vi "Tegam4040 - Close.vi"(8 "error in (no error)":errorcluster, 11 "Instrument Session Handle":u32 format="%x") -> (0 "error out":errorcluster)   [LabVIEW 2010, in "Tegam4040.lvlib"]
doc: "Closes a device session or event object specified by VISA resource name. For each VISA session that you open, you should close the session when you are finished with it. This function accepts all available classes."
uses:
  Tegam4040.lvlib
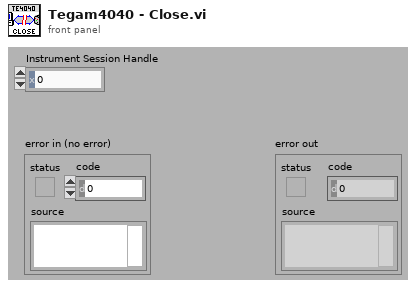
[diagram p1: front panel]
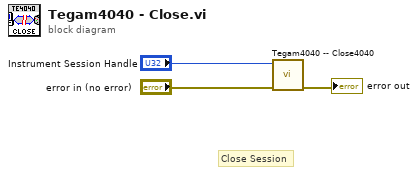
[diagram p0: block diagram]
diagram:
  # "Close Session"
  n1 = call "Tegam4040 -- Close4040.vi"("error in (no error)"="error in (no error)", "Instrument Session Handle"="Instrument Session Handle") -> ("error out"=→"error out":errorcluster)  [unwired: 9 in]
